vi "GEN_CulArray.vi"(8 "Max Values":i32, 9 "Data_Cluster":T1 {"GUI Data Cluster"."SBR" format="%08b"}) -> (1 "Data_Cluster Out":T1 {"GUI Data Cluster"."SBR" format="%08b"})   [LabVIEW 2021]
uses:
  Data_Cluster.ctl
  Measurement_Cluster.ctl
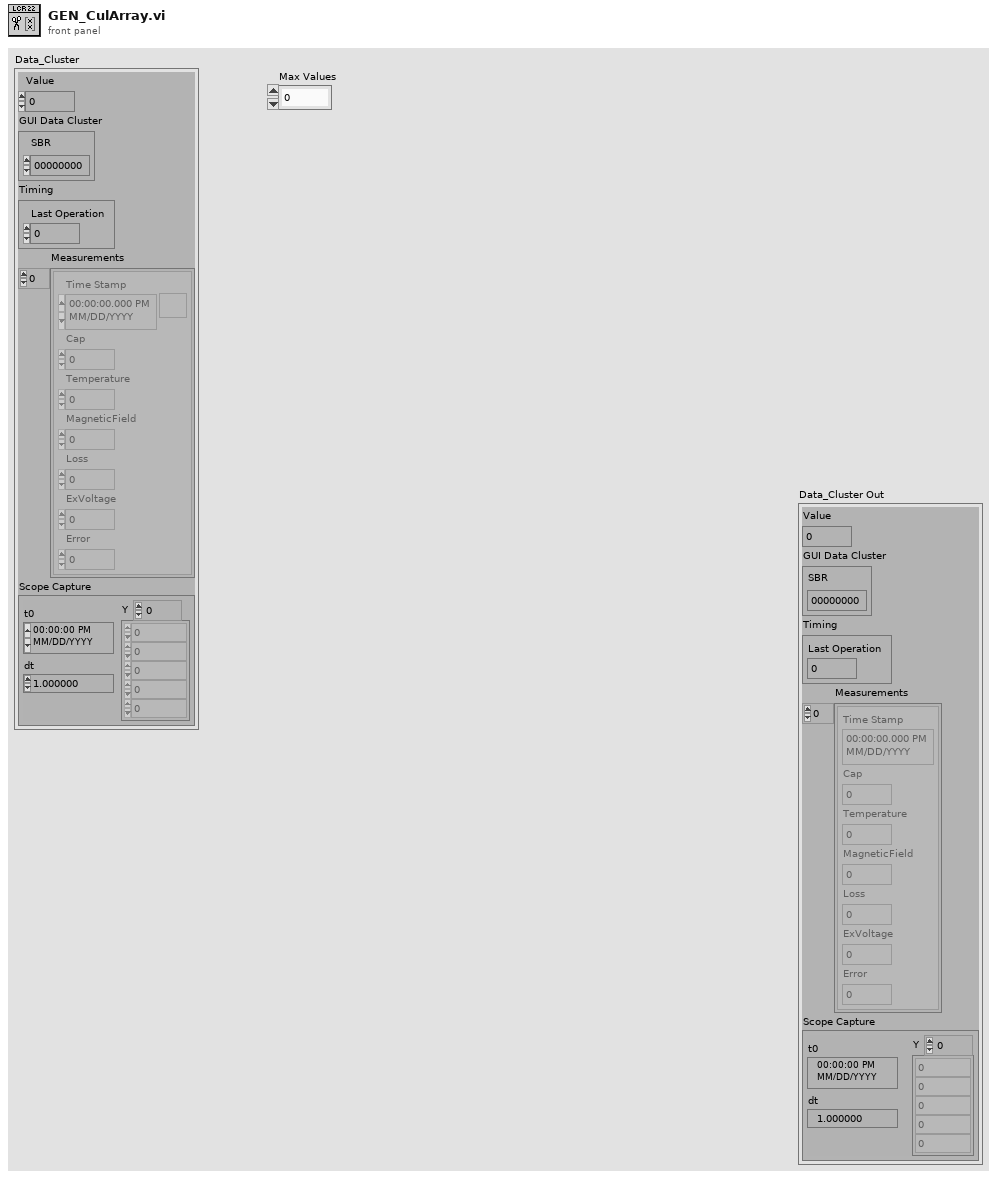
[diagram p1: front panel]
types:
  T1 = typedef "Data_Cluster.ctl" = cluster{"Value":dbl, "GUI Data Cluster":cluster{"SBR":u16}, "Timing":cluster{"Last Operation":dbl}, "Measurements":T2[], "Scope Capture":waveform(dbl)}
  T2 = typedef "Measurement_Cluster.ctl" = cluster{"Time Stamp":timestamp, "Cap":dbl, "Temperature":dbl, "MagneticField":dbl, "Loss":dbl, "ExVoltage":dbl, "Error":dbl}
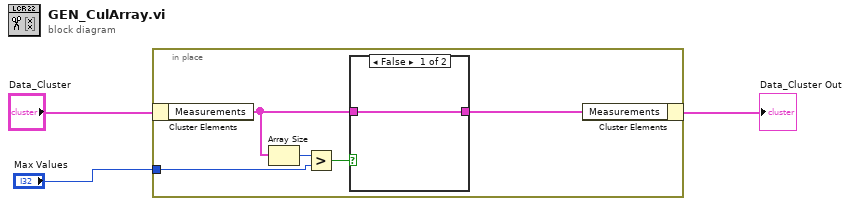
[diagram p0: block diagram]
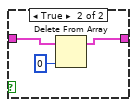
[diagram p2: hidden frame]
diagram:
  n1 = in-place {
    in-place-border: "Max Values" -> [w7]
    n2 = in-place-cluster #1("Data_Cluster") -> ("Measurements"=w5:T2[])
    n3 = Array Size(array=w5) -> (size(s)=w8:i32)
    n4 = Greater?(x=w8, y=w7) -> (0:w6:bool)
    n5 = case shown="False" w6 {
      tunnel: w5 -> [w9 w12]
      tunnel: [w9 w11] -> w4
      frame False {
      }
      frame True {
        n6 = Delete From Array(array=w12, index=0) -> (array with subset deleted=w11:T2[])  [unwired: 1 in, 1 out]
      }
    }
    n7 = in-place-cluster #1("Measurements"=w4) -> (→"Data_Cluster Out":T1)
  }
